vi "switch_capacitor.vi"(0 "Node":string, 1 "event time":string="045", 2 "Event type":string="CL", 3 "Fault type (phases)":string="BC") -> (7 "Event switches":string caption="Result")   [LabVIEW 2020]
panel:
  in  "Evento?":bool
  # "CHAVEAMENTO DE BANCO CAPACITOR\nPOR FASES (A, B, C ou combinações)"
  # "E se não encontrar a fase?\nNão vai fazer nada! simulação SEM evento"
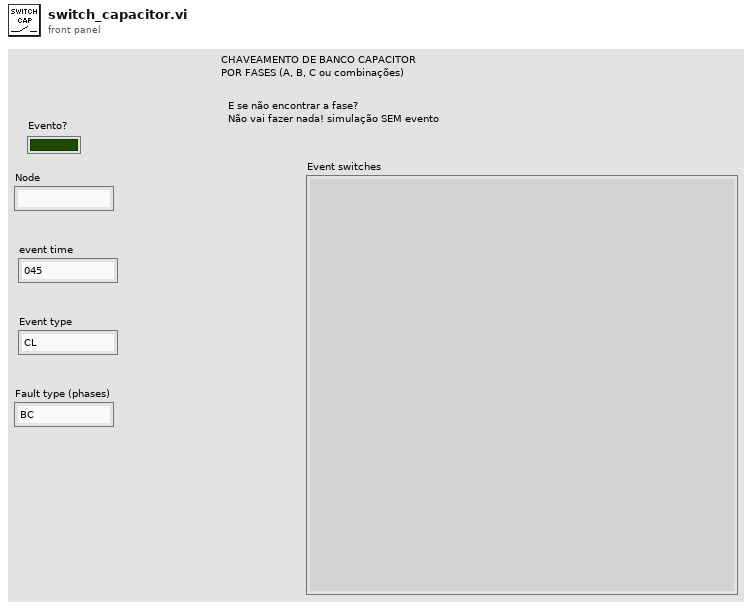
[diagram p1: front panel]
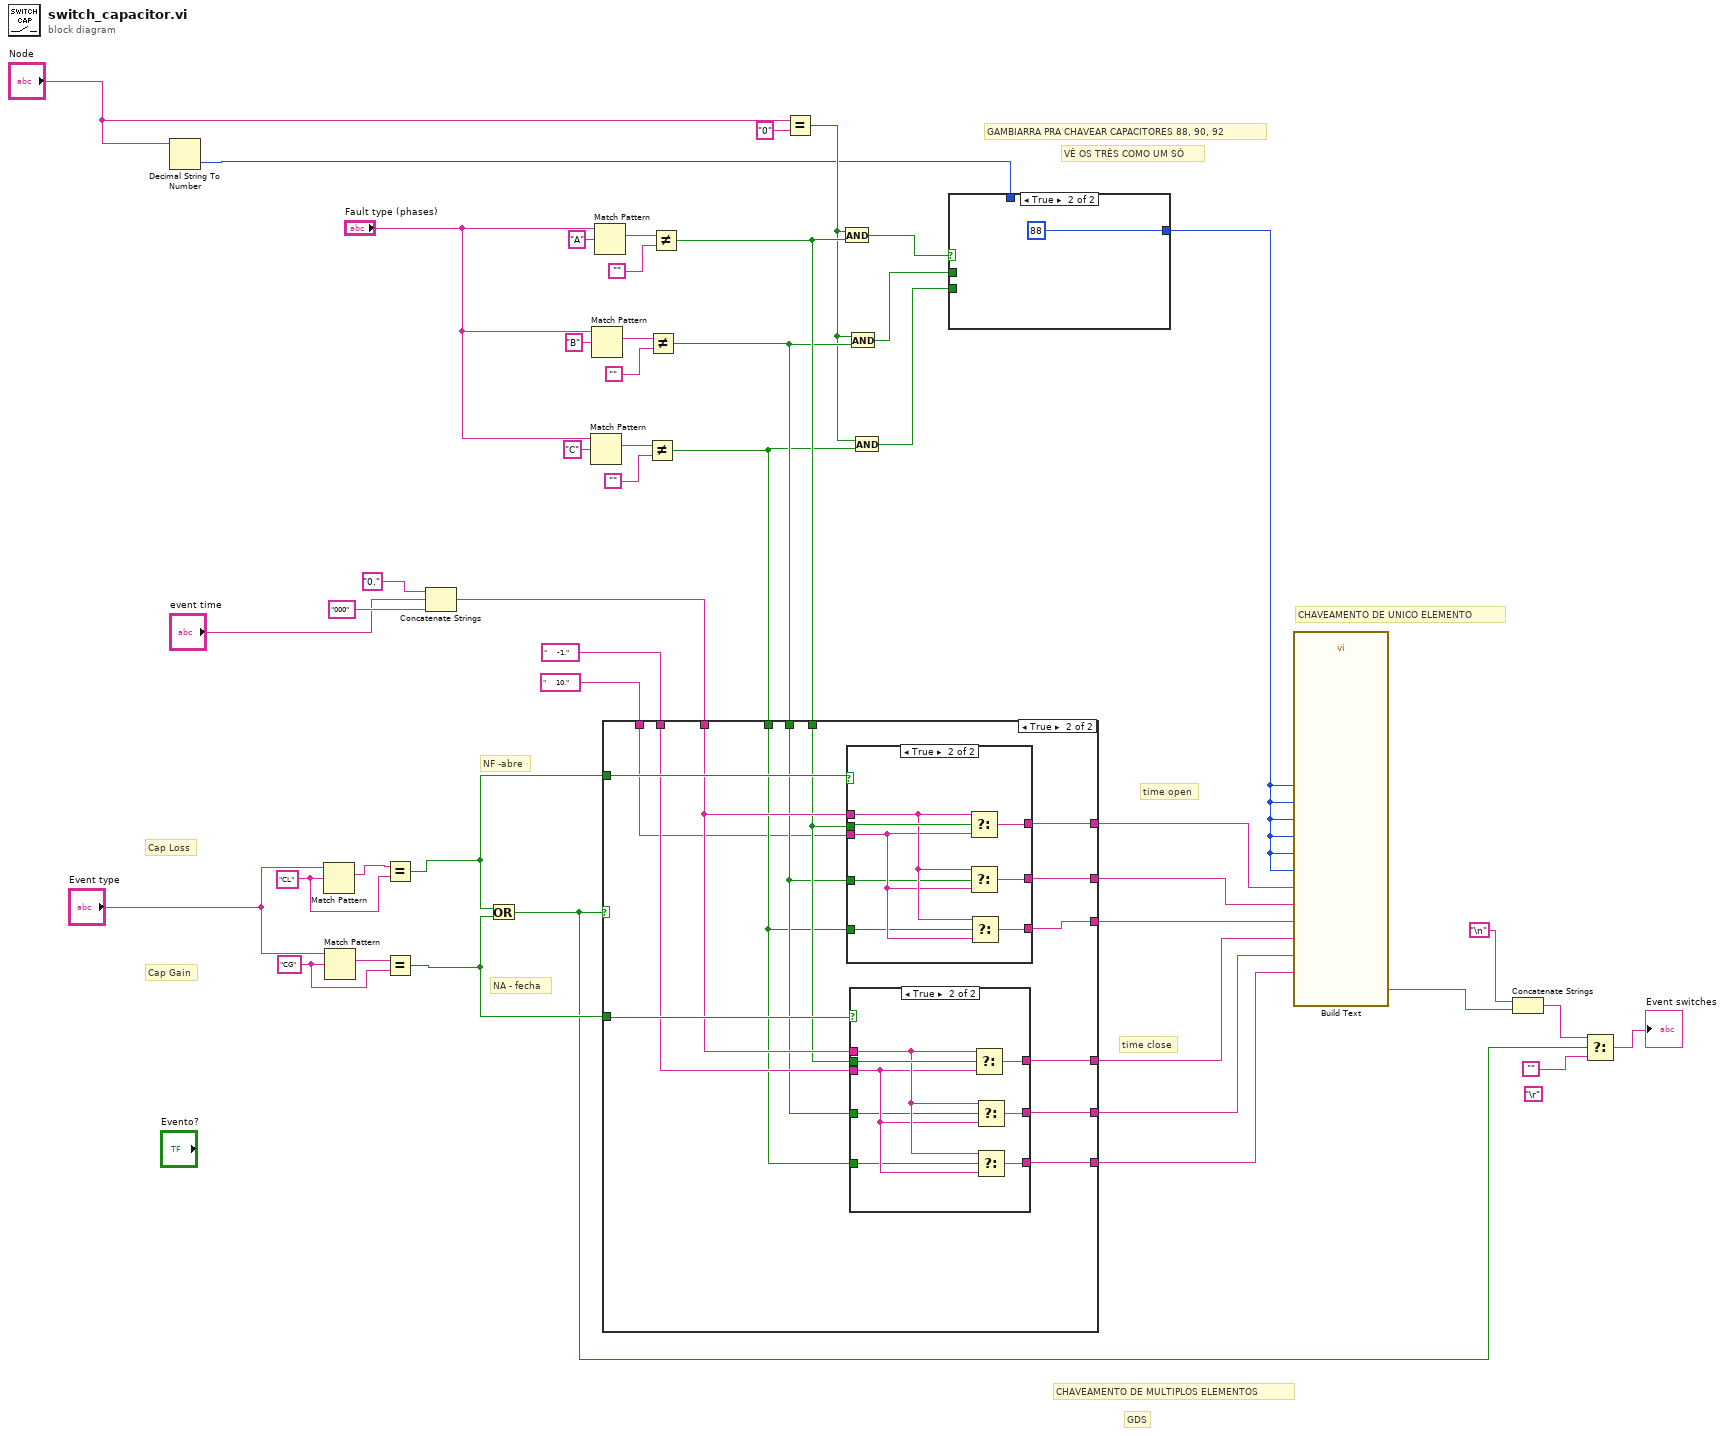
[diagram p0: block diagram]
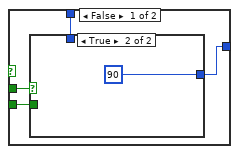
[diagram p2: hidden frame]
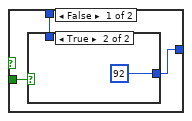
[diagram p3: hidden frame]
diagram:
  (unwired) "\r"
  w41 = "CL" ("regular expression")
  w42 = "CG" ("regular expression")
  # "VÊ OS TRÊS COMO UM SÓ"
  # "GAMBIARRA PRA CHAVEAR CAPACITORES 88, 90, 92"
  # "time close"
  # "time open"
  # "GDS"
  # "CHAVEAMENTO DE MULTIPLOS ELEMENTOS"
  # "CHAVEAMENTO DE UNICO ELEMENTO"
  # "NA - fecha"
  # "NF -abre"
  # "Cap Gain"
  # "Cap Loss"
  n1 = Decimal String To Number(string="Node") -> (number=w1:i32)  [unwired: 2 in, 1 out]
  n2 = Match Pattern(string="Event type", regular expression=w41) -> (match substring=w40:string)  [unwired: 1 in, 3 out]
  n3 = Match Pattern(string="Event type", regular expression=w42) -> (match substring=w44:string)  [unwired: 1 in, 3 out]
  n4 = Equal?(x=w40, y=w41) -> (x = y?=w35:bool)
  n5 = Equal?(x=w44, y=w42) -> (x = y?=w34:bool)
  n6 = Concatenate Strings("0." ("string"), "event time", "000" ("string")) -> (w36:string)
  n7 = Or(x=w35, y=w34) -> (x .or. y?=w33:bool)
  n8 = Match Pattern(string="Fault type (phases)", regular expression="C") -> (match substring=w23:string)  [unwired: 1 in, 3 out]
  n9 = Match Pattern(string="Fault type (phases)", regular expression="B") -> (match substring=w26:string)  [unwired: 1 in, 3 out]
  n10 = Match Pattern(string="Fault type (phases)", regular expression="A") -> (match substring=w29:string)  [unwired: 1 in, 3 out]
  n11 = Not Equal?(x=w23, y="") -> (x != y?=w9:bool)
  n12 = Not Equal?(x=w26, y="") -> (x != y?=w10:bool)
  n13 = Not Equal?(x=w29, y="") -> (x != y?=w11:bool)
  n14 = case shown="True" w33 {
    tunnel: w36 -> [_ w56]
    tunnel: "     -1." -> [w47 w57]
    tunnel: "     10." -> [w48 w49]
    tunnel: [w47 w55] -> w20
    tunnel: [w48 w62] -> w19
    tunnel: w34 -> [_ w58]
    tunnel: w35 -> [_ w61]
    tunnel: w11 -> [_ w54]
    tunnel: [w48 w60] -> w17
    tunnel: [w48 w59] -> w18
    tunnel: w10 -> [_ w53]
    tunnel: w9 -> [_ w52]
    tunnel: [w47 w51] -> w16
    tunnel: [w47 w50] -> w15
    frame False {
    }
    frame True {
      n15 = case shown="True" w61 {
        tunnel: [w72 w80] -> w62
        tunnel: w56 -> [_ w77]
        tunnel: w49 -> [w72 w76]
        tunnel: w54 -> [_ w79]
        tunnel: [w72 w78] -> w59
        tunnel: [w72 w75] -> w60
        tunnel: w53 -> [_ w74]
        tunnel: w52 -> [_ w73]
        frame False {
        }
        frame True {
          n16 = Select(t=w77, s=w79, f=w76) -> (s? t:f=w80:string)
          n17 = Select(t=w77, s=w74, f=w76) -> (s? t:f=w78:string)
          n18 = Select(t=w77, s=w73, f=w76) -> (s? t:f=w75:string)
        }
      }
      n19 = case shown="True" w58 {
        tunnel: w57 -> [w63 w68]
        tunnel: w56 -> [_ w69]
        tunnel: [w63 w71] -> w55
        tunnel: w54 -> [_ w70]
        tunnel: w53 -> [_ w67]
        tunnel: w52 -> [_ w66]
        tunnel: [w63 w65] -> w51
        tunnel: [w63 w64] -> w50
        frame False {
        }
        frame True {
          n20 = Select(t=w69, s=w70, f=w68) -> (s? t:f=w71:string)
          n21 = Select(t=w69, s=w67, f=w68) -> (s? t:f=w65:string)
          n22 = Select(t=w69, s=w66, f=w68) -> (s? t:f=w64:string)
        }
      }
    }
  }
  n23 = Equal?(x="Node", y="0") -> (x = y?=w6:bool)
  n24 = And(x=w6, y=w11) -> (x .and. y?=w5:bool)
  n25 = And(x=w6, y=w10) -> (x .and. y?=w4:bool)
  n26 = And(x=w6, y=w9) -> (x .and. y?=w3:bool)
  n27 = case shown="True" w5 {
    tunnel: [w82 88] -> w2
    tunnel: w4 -> [w84 _]
    tunnel: w3 -> [w83 _]
    tunnel: w1 -> [w81 _]
    frame False {
      n28 = case shown="True" w84 {
        tunnel: w83 -> [w87 _]
        tunnel: [w85 90] -> w82
        tunnel: w81 -> [w86 _]
        frame False {
          n29 = case shown="True" w87 {
            tunnel: [w88 92] -> w85
            tunnel: w86 -> [w88 _]
            frame False {
            }
            frame True {
            }
          }
        }
        frame True {
        }
      }
    }
    frame True {
    }
  }
  n30 = call "Build Text"("inA"=w2, "inA_2"=w2, "time_close_A"=w20, "time_open_A"=w19, "inB"=w2, "inB_2"=w2, "time_close_B"=w16, "time_open_B"=w18, "inC"=w2, "inC_2"=w2, "time_close_C"=w15, "time_open_C"=w17) -> ("Result"=w13:string)  [unwired: 14 in, 1 out]
  n31 = Concatenate Strings("\n", w13) -> (w31:string)
  n32 = Select(t=w31, s=w33, f="") -> (s? t:f=→"Event switches":string)
